vi "Get Job Attributes Boolean.vi"(10 "element":string, 11 "JOB Attributes":string[][](array[string])) -> (3 "Cell Value":bool)   [LabVIEW 2021]
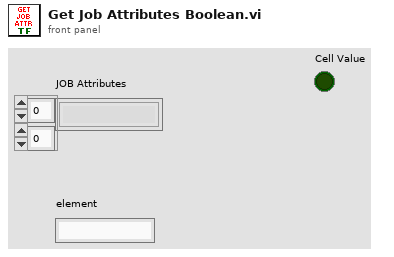
[diagram p1: front panel]
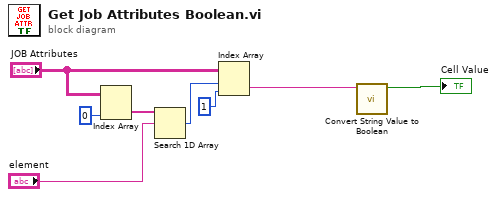
[diagram p0: block diagram]
diagram:
  n1 = Index Array(array="JOB Attributes", index (col)=0 ("disabled index (col)")) -> (element=w4:string[])  [unwired: 1 in]
  n2 = Search 1D Array(1D array=w4, element="element") -> (index of element=w7:i32)  [unwired: 1 in]
  n3 = Index Array(array="JOB Attributes", index (row)=w7, index (col)=1 ("disabled index (col)")) -> (element=w2:string)
  n4 = call "Convert String Value to Boolean.vi"("Cell String"=w2) -> ("Boolean"=→"Cell Value":bool)  [unwired: 10 in]
